vi "StellarNet Init & Count.vi"(8 "error in":errorcluster) -> (0 "error out":errorcluster, 3 "Number of Channels":i32)   [LabVIEW 2020]
uses:
  Swdll.dll
panel:
  # "This subVI initializes the .dll and returns the number of attached spectrometers found by the .dll"
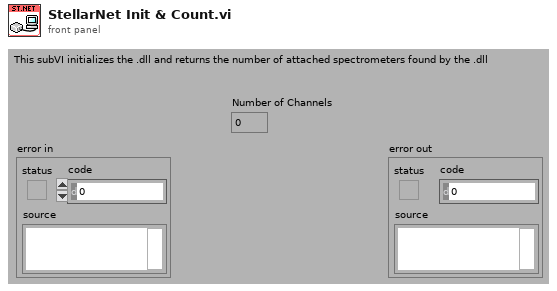
[diagram p1: front panel]
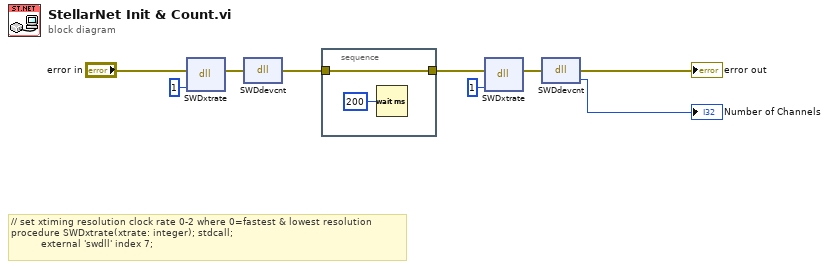
[diagram p0: block diagram]
diagram:
  # "// set xtiming resolution clock rate 0-2 where 0=fastest & lowest resolution\nprocedure SWDxtrate(xtrate: integer); stdcall;\n          external 'swdll' index 7;"
  n1 = dll-call lib="C:/GEECS/Developers Version/source/Device Drivers/StellarNet Black-Comet Spectrometer/SupportLib/InstrumentsComm/Swdll.dll" fn="SWDxtrate" label="xtrate"(error in="error in", "xtrate"=1) -> (error out=w8:errorcluster)  [unwired: 4 in, 1 out]
  n2 = dll-call lib="C:/GEECS/Developers Version/source/Device Drivers/StellarNet Black-Comet Spectrometer/SupportLib/InstrumentsComm/swdll.dll" fn="SWDdevcnt"(error in=w8) -> (error out=w6:errorcluster)  [unwired: 3 in, 1 out]
  n3 = stacked-sequence {
    tunnel: w6 -> [w10]
    tunnel: [w10] -> w3
    frame #0 {
      n4 = Wait (ms)(milliseconds to wait=u32 200) -> ()  [unwired: 1 out]
    }
  }
  n5 = dll-call lib="C:/GEECS/Developers Version/source/Device Drivers/StellarNet Black-Comet Spectrometer/SupportLib/InstrumentsComm/Swdll.dll" fn="SWDxtrate" label="xtrate"(error in=w3, "xtrate"=1) -> (error out=w5:errorcluster)  [unwired: 4 in, 1 out]
  n6 = dll-call lib="C:/GEECS/Developers Version/source/Device Drivers/StellarNet Black-Comet Spectrometer/SupportLib/InstrumentsComm/swdll.dll" fn="SWDdevcnt"(error in=w5) -> (error out=→"error out":errorcluster, "NumChan"=→"Number of Channels":i32)  [unwired: 2 in, 1 out]
